vi "oa_SCL Draw Axes.vi"(5 "[user-specified font]":T4, 7 "desired font(Application)":T3(ring)=enum."Application Font", 8 "grid cosmetics":T2={"line color"=39168, "text color"=65280, "tick length"=3, "crossing axes"=FALSE, "visible grid?"=TRUE}, 9 "y axis attributes":T1={"coordinate 1"=0, "value 1"=0.0, "coordinate 2"=0, "value 2"=0.0, "log?"=FALSE, "fmt and prec"={"format"=enum."Decimal", "precision"=2}} {"value 2" format="%.2f"; "value 1" format="%.2f"}, 10 "x axis attributes":T1={"coordinate 1"=0, "value 1"=0.0, "coordinate 2"=0, "value 2"=0.0, "log?"=FALSE, "fmt and prec"={"format"=enum."Decimal", "precision"=2}} {"value 2" format="%.2f"; "value 1" format="%.2f"}, 11 "picture":picture) -> (1 "y scale specs":cluster{"coordinate":i16, "label":string}[](array[cluster]), 2 "x scale specs":cluster{"coordinate":i16, "label":string}[](array[cluster]), 3 "new picture":picture)   [LabVIEW 2017]
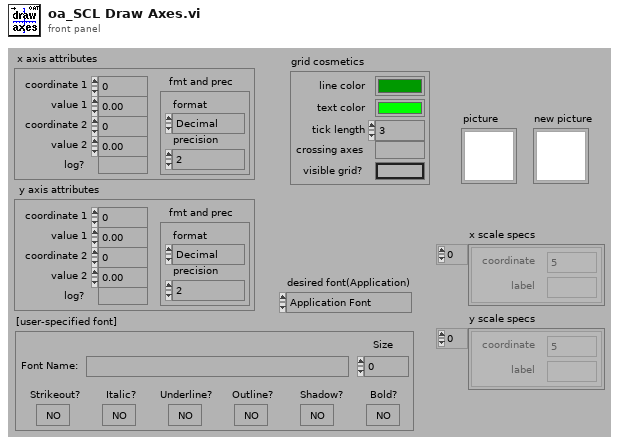
[diagram p1: front panel]
types:
  T1 = cluster{"coordinate 1":i16, "value 1":dbl, "coordinate 2":i16, "value 2":dbl, "log?":bool, "fmt and prec":cluster{"format":enum8{"Decimal", "Scientific", "Engineering", "Binary", "Octal", "Hex"}, "precision":u8}}
  T2 = cluster{"line color":u32, "text color":u32, "tick length":i16, "crossing axes":bool, "visible grid?":bool}
  T3 = enum16{"User-specified Font", "Application Font", "System Font", "Dialog Font"}
  T4 = cluster{"Font Name:":string, "Size":i16, "Strikeout?":bool, "Italic?":bool, "Underline?":bool, "Outline?":bool, "Shadow?":bool, "Bold?":bool}
  T5 = cluster{bool, bool, bool, "line color":u32, "text color":u32}
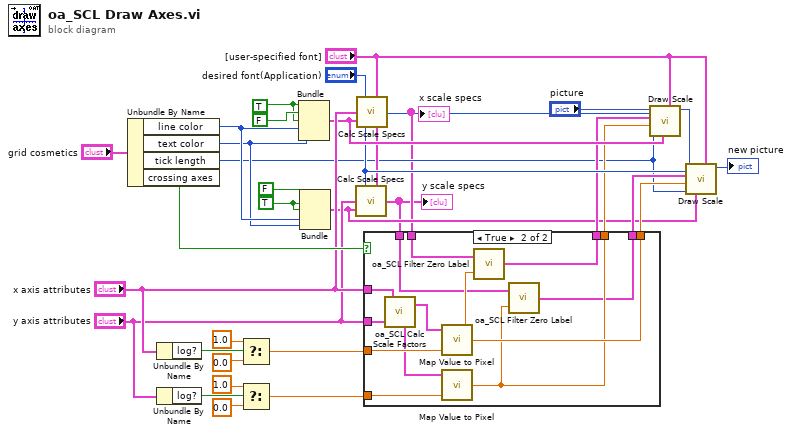
[diagram p0: block diagram]
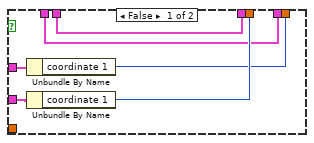
[diagram p2: hidden frame]
diagram:
  w3 = TRUE
  w1 = TRUE
  n1 = Unbundle By Name("grid cosmetics") -> ("line color"=w19:u32, "text color"=w18:u32, "tick length"=w17:i16, "crossing axes"=w32:bool)
  n2 = Unbundle By Name("x axis attributes") -> ("log?"=w8:bool)
  n3 = Unbundle By Name("y axis attributes") -> ("log?"=w13:bool)
  n4 = Select(t=1.0, s=w8, f=0.0) -> (s? t:f=w7:dbl)
  n5 = Select(t=1.0, s=w13, f=0.0) -> (s? t:f=w14:dbl)
  n6 = Bundle(w1, FALSE, w1, "line color"=w19, "text color"=w18) -> (w30:T5)  [unwired: 1 in]
  n7 = Bundle(FALSE, w3, w3, "line color"=w19, "text color"=w18) -> (w11:T5)  [unwired: 1 in]
  n8 = call <vilib>:"Calc Scale Specs.vi"("desired font(Application)"="desired font(Application)", "scale definition"="y axis attributes", "scale attributes"=w11, "[user-specified font]"="[user-specified font]") -> ("scale specs"=w5:cluster{"coordinate":i16, "label":string}[])  [unwired: 5 in]
  "y scale specs" <- w5
  n9 = call <vilib>:"Calc Scale Specs.vi"("desired font(Application)"="desired font(Application)", "scale definition"="x axis attributes", "scale attributes"=w30, "[user-specified font]"="[user-specified font]") -> ("scale specs"=w6:cluster{"coordinate":i16, "label":string}[])  [unwired: 5 in]
  "x scale specs" <- w6
  n10 = case shown="True" w32 {
    tunnel: "x axis attributes" -> [w36 w40]
    tunnel: "y axis attributes" -> [w37 w39]
    tunnel: w5 -> [w35 w46]
    tunnel: w6 -> [w34 w50]
    tunnel: [w35 w45] -> w26
    tunnel: [w34 w48] -> w28
    tunnel: [w33 w49] -> w25
    tunnel: [w38 w47] -> w27
    tunnel: w14 -> [_ w44]
    tunnel: w7 -> [_ w43]
    frame False {
      n11 = Unbundle By Name(w36) -> ("coordinate 1"=w33:i16)
      n12 = Unbundle By Name(w37) -> ("coordinate 1"=w38:i16)
    }
    frame True {
      n13 = call <vilib>:"oa_SCL Calc Scale Factors.vi"("y axis attributes"=w39, "x axis attributes"=w40) -> ("y scale factors"=w42:cluster{"a":dbl, "b":dbl, "log?":bool}, "x scale factors"=w41:cluster{"a":dbl, "b":dbl, "log?":bool})
      n14 = call <vilib>:"Map Value to Pixel.vi"("x"=w43, "scale factors"=w41) -> ("pixel"=w49:dbl)  [unwired: 1 in]
      n15 = call <vilib>:"Map Value to Pixel.vi"("x"=w44, "scale factors"=w42) -> ("pixel"=w47:dbl)  [unwired: 1 in]
      n16 = call <vilib>:"oa_SCL Filter Zero Label.vi"("zero coordinate"=w49, "scale specs 2"=w50) -> ("scale specs"=w48:cluster{"coordinate":i16, "label":string}[])
      n17 = call <vilib>:"oa_SCL Filter Zero Label.vi"("zero coordinate"=w47, "scale specs 2"=w46) -> ("scale specs"=w45:cluster{"coordinate":i16, "label":string}[])
    }
  }
  n18 = call <vilib>:"Draw Scale.vi"("[user-specified font]"="[user-specified font]", "scale attributes"=w30, "desired font(Application)"="desired font(Application)", "tick length(3)"=w17, "constant coordinate"=w27, "scale specs"=w28, "picture"="picture") -> ("new picture"=w23:picture)  [unwired: 4 in]
  n19 = call <vilib>:"Draw Scale.vi"("[user-specified font]"="[user-specified font]", "scale attributes"=w11, "desired font(Application)"="desired font(Application)", "tick length(3)"=w17, "constant coordinate"=w25, "scale specs"=w26, "picture"=w23) -> ("new picture"=→"new picture":picture)  [unwired: 4 in]
